vi "Waveform Parameters 2.vi"(11 "Test No":T1) -> (0 "Active/Passive Holdoff  (µs)":dbl[](array[numeric])=[1.0, 15000.0, 200.0, 1.0, 15000.0, 100.0], 1 "Active/Passive Recovery PW (µs)":dbl[](array[numeric])=[15000.0, 10.0, 300.0, 15000.0, 10.0, 75.0], 2 "Active Recovery Amp (mA)":dbl[](array[numeric])=[1.0, 255.0, 100.0, 1.0, 255.0, 100.0], 3 "Interphase Delay (µs)":dbl[](array[numeric])=[1.0, 255.0, 100.0, 1.0, 255.0, 100.0], 4 "CBC width (µs)":dbl[](array[numeric])=[2000.0, 10000.0, 400.0, 1.0, 10000.0, 50.0], 5 "Stim Pulse Width (µs)":dbl[](array[numeric])=[10.0, 1500.0, 500.0, 10.0, 1500.0, 100.0], 6 "CBC Holdoff (µs)":dbl[](array[numeric])=[1.0, 15000.0, 600.0, 1.0, 15000.0, 100.0], 7 "Stim Amplitude (mA)":dbl[](array[numeric])=[-15.0, -0.015, -5.0, 15.0, 0.015, 3.0], 8 "Frequency (Hz)":dbl[](array[numeric])=[2.0, 22.0, 170.0, 2.0, 18.0, 170.0], 9 "Frequency Index":dbl[](array[numeric])=[0.0, 11.0, 36.0, 0.0, 9.0, 36.0], 10 "Sample Rate(Samples/sec)":dbl[](array[numeric])=[2000.0, 22000.0, 170000.0, 2000.0, 18000.0, 170000.0])   [LabVIEW 2010]
uses:
  Waveform Parameters Test No.ctl
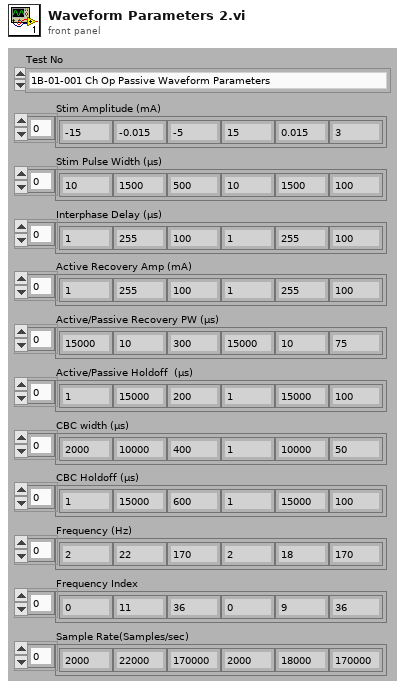
[diagram p1: front panel]
types:
  T1 = typedef "Waveform Parameters Test No.ctl" = enum16{"1B-01-001 Ch Op Passive Waveform Parameters", "1B-01-002 Enclosure Op Passive Waveform Parameters", "1B-01-003 Ch Op Active Waveform Parameters", "1B-01-004 Enclosure Op Active Waveform Parameters"}
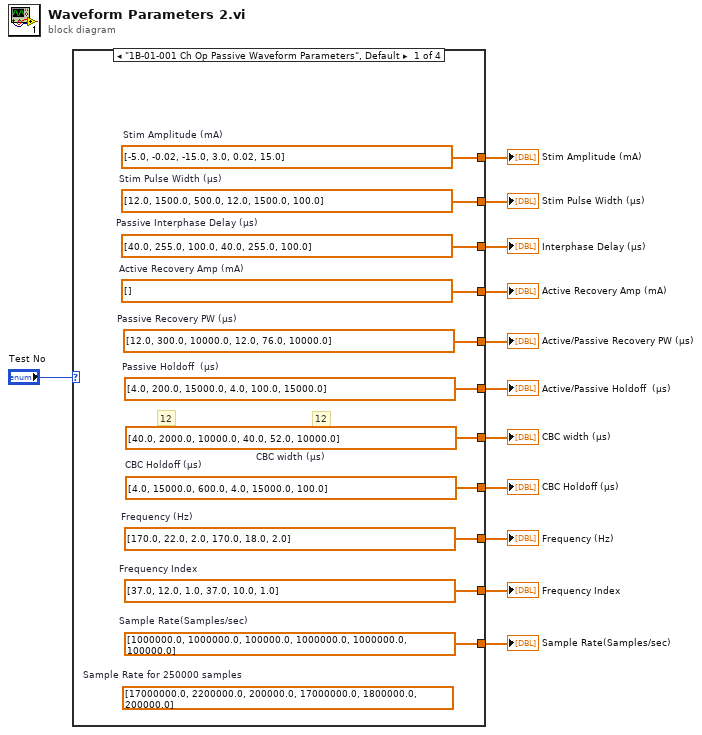
[diagram p0: block diagram]
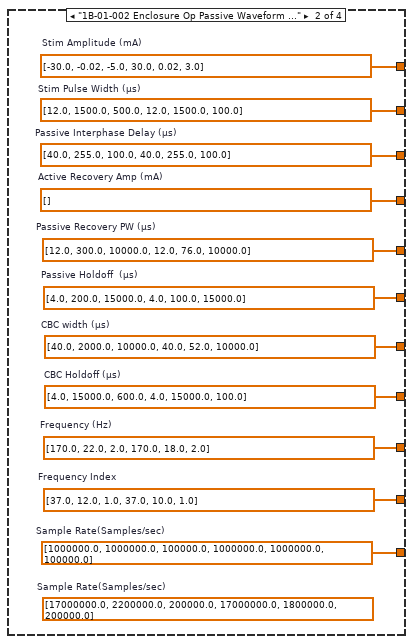
[diagram p2: hidden frame]
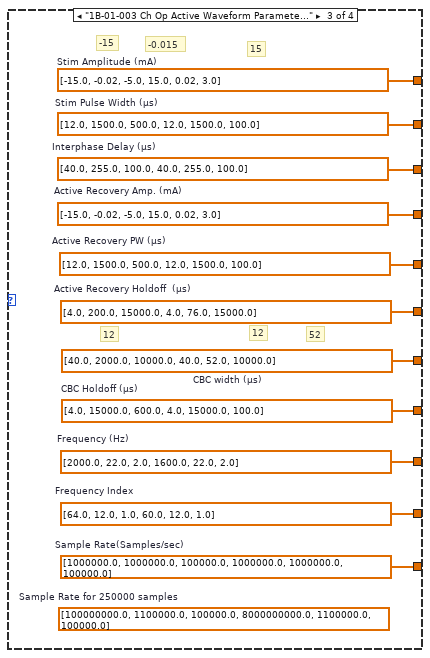
[diagram p3: hidden frame]
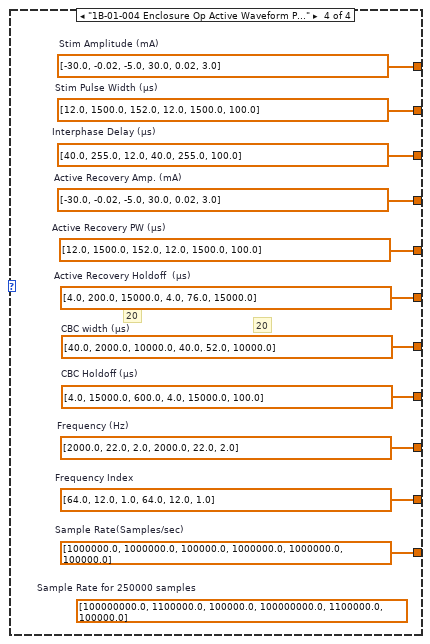
[diagram p4: hidden frame]
diagram:
  n1 = case shown="\"1B-01-001 Ch Op Passive Waveform Parameters\", Default" "Test No" {
    tunnel: [w23 w34 w45 w56] -> w12
    tunnel: [w22 w33 w44 w55] -> w11
    tunnel: [w21 w32 w43 w54] -> w10
    tunnel: [w20 w31 w42 w53] -> w9
    tunnel: [w19 w30 w41 w52] -> w8
    tunnel: [w18 w29 w40 w51] -> w7
    tunnel: [w17 w28 w39 w50] -> w6
    tunnel: [w16 w27 w38 w49] -> w5
    tunnel: [w15 w26 w37 w48] -> w4
    tunnel: [w14 w24 w36 w47] -> w3
    tunnel: [w13 w25 w35 w46] -> w1
    frame "1B-01-001 Ch Op Passive Waveform Parameters", Default {
      (unwired) dbl[] [17000000.0, 2200000.0, 200000.0, 17000000.0, 1800000.0, 200000.0]  # Sample Rate for 250000 samples
      w13 = dbl[] []  # Active Recovery Amp (mA)
      w14 = dbl[] [1000000.0, 1000000.0, 100000.0, 1000000.0, 1000000.0, 100000.0]  # Sample Rate(Samples/sec)
      w15 = dbl[] [37.0, 12.0, 1.0, 37.0, 10.0, 1.0]  # Frequency Index
      w16 = dbl[] [170.0, 22.0, 2.0, 170.0, 18.0, 2.0]  # Frequency (Hz)
      w17 = dbl[] [4.0, 15000.0, 600.0, 4.0, 15000.0, 100.0]  # CBC Holdoff (µs)
      w18 = dbl[] [40.0, 2000.0, 10000.0, 40.0, 52.0, 10000.0]  # CBC width (µs)
      w19 = dbl[] [4.0, 200.0, 15000.0, 4.0, 100.0, 15000.0]  # Passive Holdoff  (µs)
      w20 = dbl[] [12.0, 300.0, 10000.0, 12.0, 76.0, 10000.0]  # Passive Recovery PW (µs)
      w21 = dbl[] [40.0, 255.0, 100.0, 40.0, 255.0, 100.0]  # Passive Interphase Delay (µs)
      w22 = dbl[] [12.0, 1500.0, 500.0, 12.0, 1500.0, 100.0]  # Stim Pulse Width (µs)
      w23 = dbl[] [-5.0, -0.02, -15.0, 3.0, 0.02, 15.0]  # Stim Amplitude (mA)
      # "12"
      # "12"
    }
    frame "1B-01-002 Enclosure Op Passive Waveform Parameters" {
      (unwired) dbl[] [17000000.0, 2200000.0, 200000.0, 17000000.0, 1800000.0, 200000.0]  # Sample Rate(Samples/sec)
      w24 = dbl[] [1000000.0, 1000000.0, 100000.0, 1000000.0, 1000000.0, 100000.0]  # Sample Rate(Samples/sec)
      w25 = dbl[] []  # Active Recovery Amp (mA)
      w26 = dbl[] [37.0, 12.0, 1.0, 37.0, 10.0, 1.0]  # Frequency Index
      w27 = dbl[] [170.0, 22.0, 2.0, 170.0, 18.0, 2.0]  # Frequency (Hz)
      w28 = dbl[] [4.0, 15000.0, 600.0, 4.0, 15000.0, 100.0]  # CBC Holdoff (µs)
      w29 = dbl[] [40.0, 2000.0, 10000.0, 40.0, 52.0, 10000.0]  # CBC width (µs)
      w30 = dbl[] [4.0, 200.0, 15000.0, 4.0, 100.0, 15000.0]  # Passive Holdoff  (µs)
      w31 = dbl[] [12.0, 300.0, 10000.0, 12.0, 76.0, 10000.0]  # Passive Recovery PW (µs)
      w32 = dbl[] [40.0, 255.0, 100.0, 40.0, 255.0, 100.0]  # Passive Interphase Delay (µs)
      w33 = dbl[] [12.0, 1500.0, 500.0, 12.0, 1500.0, 100.0]  # Stim Pulse Width (µs)
      w34 = dbl[] [-30.0, -0.02, -5.0, 30.0, 0.02, 3.0]  # Stim Amplitude (mA)
    }
    frame "1B-01-003 Ch Op Active Waveform Parameters" {
      (unwired) dbl[] [100000000.0, 1100000.0, 100000.0, 8000000000.0, 1100000.0, 100000.0]  # Sample Rate for 250000 samples
      w35 = dbl[] [-15.0, -0.02, -5.0, 15.0, 0.02, 3.0]  # Active Recovery Amp. (mA)
      w36 = dbl[] [1000000.0, 1000000.0, 100000.0, 1000000.0, 1000000.0, 100000.0]  # Sample Rate(Samples/sec)
      w37 = dbl[] [64.0, 12.0, 1.0, 60.0, 12.0, 1.0]  # Frequency Index
      w38 = dbl[] [2000.0, 22.0, 2.0, 1600.0, 22.0, 2.0]  # Frequency (Hz)
      w39 = dbl[] [4.0, 15000.0, 600.0, 4.0, 15000.0, 100.0]  # CBC Holdoff (µs)
      w40 = dbl[] [40.0, 2000.0, 10000.0, 40.0, 52.0, 10000.0]  # CBC width (µs)
      w41 = dbl[] [4.0, 200.0, 15000.0, 4.0, 76.0, 15000.0]  # Active Recovery Holdoff  (µs)
      w42 = dbl[] [12.0, 1500.0, 500.0, 12.0, 1500.0, 100.0]  # Active Recovery PW (µs)
      w43 = dbl[] [40.0, 255.0, 100.0, 40.0, 255.0, 100.0]  # Interphase Delay (µs)
      w44 = dbl[] [12.0, 1500.0, 500.0, 12.0, 1500.0, 100.0]  # Stim Pulse Width (µs)
      w45 = dbl[] [-15.0, -0.02, -5.0, 15.0, 0.02, 3.0]  # Stim Amplitude (mA)
      # "52"
      # "12"
      # "12"
      # "-0.015"
      # "15"
      # "-15"
    }
    frame "1B-01-004 Enclosure Op Active Waveform Parameters" {
      (unwired) dbl[] [100000000.0, 1100000.0, 100000.0, 100000000.0, 1100000.0, 100000.0]  # Sample Rate for 250000 samples
      w46 = dbl[] [-30.0, -0.02, -5.0, 30.0, 0.02, 3.0]  # Active Recovery Amp. (mA)
      w47 = dbl[] [1000000.0, 1000000.0, 100000.0, 1000000.0, 1000000.0, 100000.0]  # Sample Rate(Samples/sec)
      w48 = dbl[] [64.0, 12.0, 1.0, 64.0, 12.0, 1.0]  # Frequency Index
      w49 = dbl[] [2000.0, 22.0, 2.0, 2000.0, 22.0, 2.0]  # Frequency (Hz)
      w50 = dbl[] [4.0, 15000.0, 600.0, 4.0, 15000.0, 100.0]  # CBC Holdoff (µs)
      w51 = dbl[] [40.0, 2000.0, 10000.0, 40.0, 52.0, 10000.0]  # CBC width (µs)
      w52 = dbl[] [4.0, 200.0, 15000.0, 4.0, 76.0, 15000.0]  # Active Recovery Holdoff  (µs)
      w53 = dbl[] [12.0, 1500.0, 152.0, 12.0, 1500.0, 100.0]  # Active Recovery PW (µs)
      w54 = dbl[] [40.0, 255.0, 12.0, 40.0, 255.0, 100.0]  # Interphase Delay (µs)
      w55 = dbl[] [12.0, 1500.0, 152.0, 12.0, 1500.0, 100.0]  # Stim Pulse Width (µs)
      w56 = dbl[] [-30.0, -0.02, -5.0, 30.0, 0.02, 3.0]  # Stim Amplitude (mA)
      # "20"
      # "20"
    }
  }
  "Stim Amplitude (mA)" <- w12
  "Stim Pulse Width (µs)" <- w11
  "Interphase Delay (µs)" <- w10
  "Active/Passive Recovery PW (µs)" <- w9
  "Active/Passive Holdoff  (µs)" <- w8
  "CBC width (µs)" <- w7
  "CBC Holdoff (µs)" <- w6
  "Frequency (Hz)" <- w5
  "Frequency Index" <- w4
  "Sample Rate(Samples/sec)" <- w3
  "Active Recovery Amp (mA)" <- w1
